vi "svl_Generate Waterfall View.vi"(1 "scale info":cluster{"x scale":dbl[], "y scale":dbl[]} {"y scale" format="%.2f"; "x scale" format="%.2f"}, 2 "clipped data":dbl[][](array[numeric]) format="%.2f", 3 "dX/dY":dbl format="%.2f", 4 "dY":dbl format="%.2f", 5 "y scale":cluster{"y min":dbl, "y max":dbl} {"y max" format="%.2f"; "y min" format="%.2f"}, 6 "subset info":T1) -> (0 "waterfall view":cluster{dbl[], dbl[]}[](array[cluster]) {"?" format="%.2f"; "?" format="%.2f"})   [LabVIEW 2017]
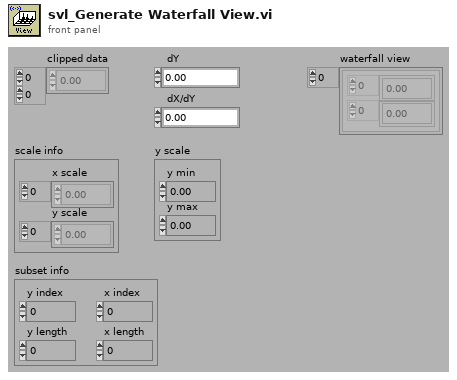
[diagram p1: front panel]
types:
  T1 = cluster{"y index":i32, "y length":i32, "x index":i32, "x length":i32}
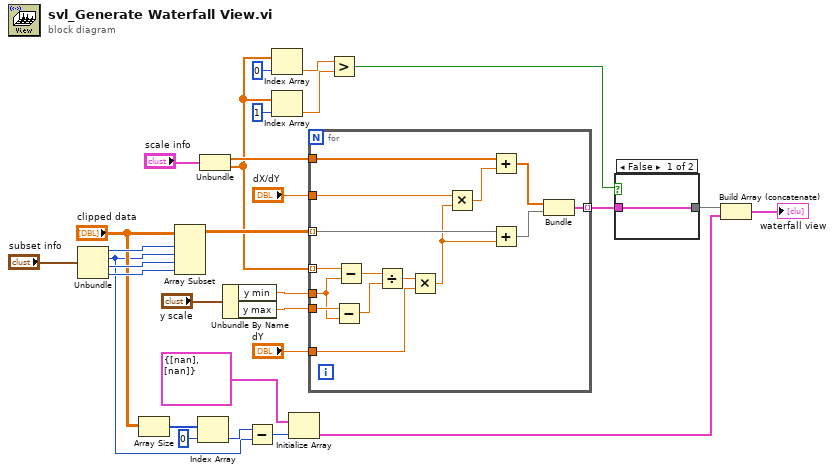
[diagram p0: block diagram]
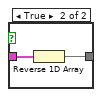
[diagram p2: hidden frame]
diagram:
  n1 = Unbundle("subset info") -> ("y index"=w19:i32, "y length"=w14:i32, "x index"=w20:i32, "x length"=w21:i32)
  n2 = Array Size(array="clipped data") -> (size(s)=w17:i32[])
  n3 = Array Subset(array="clipped data", index (row)=w19, length (row)=w14, index (col)=w20, length (col)=w21) -> (w23:dbl[][])
  n4 = Index Array(array=w17, index=0) -> (element=w15:i32)
  n5 = Unbundle("scale info") -> ("x scale"=w27:dbl[], "y scale"=w4:dbl[])
  n6 = Unbundle By Name("y scale") -> ("y min"=w25:dbl, "y max"=w24:dbl)
  n7 = Subtract(x=w15, y=w14) -> (x-y=w13:i32)
  n8 = Index Array(array=w4, index=0) -> (element=w3:dbl)
  n9 = Index Array(array=w4, index=1) -> (element=w2:dbl)
  n10 = Initialize Array(cluster{dbl[], dbl[]} {[nan], [nan]} ("frame"), w13) -> (w11:cluster{dbl[], dbl[]}[])
  n11 = for {
    tunnel: w4 -> [w44] mode=indexing
    tunnel: w24 -> [w43]
    tunnel: w25 -> [w42]
    tunnel: w23 -> [w39] mode=indexing
    tunnel: w27 -> [w36]
    tunnel: "dX/dY" -> [w34]
    tunnel: [w33] -> w8 mode=indexing
    tunnel: "dY" -> [w31]
    n12 = Subtract(x=w43, y=w42) -> (x-y=w40:dbl)
    n13 = Subtract(x=w44, y=w42) -> (x-y=w41:dbl)
    n14 = Divide(x=w41, y=w40) -> (x/y=w32:dbl)
    n15 = Multiply(x=w32, y=w31) -> (x*y=w30:dbl)
    n16 = Multiply(x=w34, y=w30) -> (x*y=w35:dbl)
    n17 = Add(x=w36, y=w35) -> (x+y=w37:dbl[])
    n18 = Add(x=w39, y=w30) -> (x+y=w38:dbl[])
    n19 = Bundle(w37, w38) -> (w33:cluster{dbl[], dbl[]})  [unwired: 1 in]
  }
  n20 = Greater?(x=w3, y=w2) -> (0:w1:bool)
  n21 = case shown="False" w1 {
    tunnel: w8 -> [w45 w47]
    tunnel: [w45 w46] -> w7
    frame False {
    }
    frame True {
      n22 = Reverse 1D Array(array=w47) -> (reversed array=w46:cluster{dbl[], dbl[]}[])
    }
  }
  n23 = Build Array (concatenate)(w7, w11) -> (→"waterfall view":cluster{dbl[], dbl[]}[])
